vi "ConvertBoolToStr.vi"(11 "bool":bool) -> (3 "result":string)   [LabVIEW 2018, in "Library-DataConvert.lvlib"]
uses:
  Library-DataConvert.lvlib
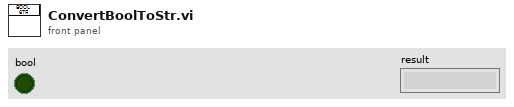
[diagram p1: front panel]
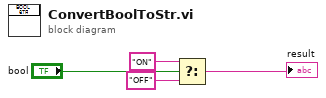
[diagram p0: block diagram]
diagram:
  n1 = Select(t="ON" ("y"), s="bool", f="OFF" ("y")) -> (s? t:f=→"result":string)
